vi "open.vi"(8 "error in (no error)":errorcluster, 11 "Scintilla window ref":refnum<k24>) -> (0 "error out":errorcluster, 3 "ScintillaNET out":refnum<class "ScintillaNET.lvclass">)   [LabVIEW 2018, in "ScintillaNET.lvclass"]
uses:
  ScintillaNET.lvclass
  D:/project/hobby/LF2R/LabVIEW/source/ScintillaNET/dll/ScintillaNET.dll
  dll/ScintillaNET.dll
  ScintillaNET.lvclass/ScintillaNET.ctl
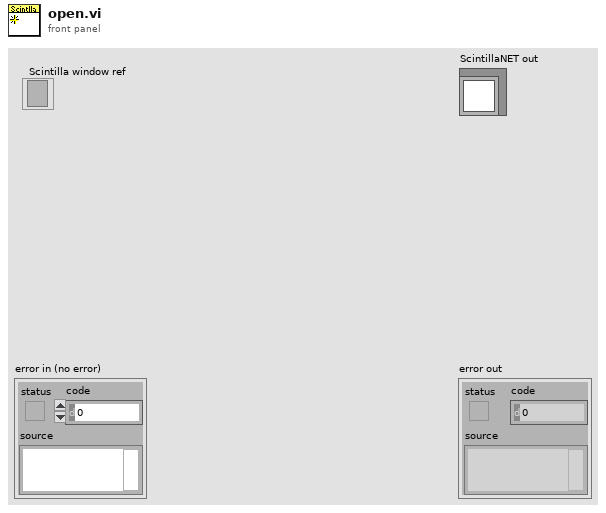
[diagram p1: front panel]
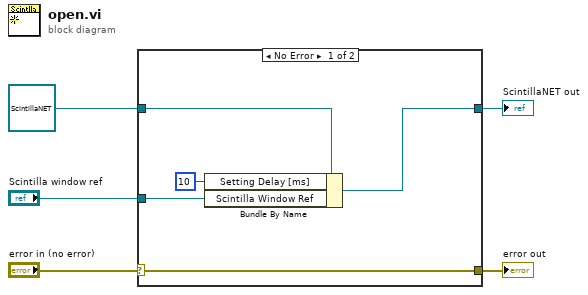
[diagram p0: block diagram]
diagram:
  n1 = case shown="No Error" "error in (no error)" {
    selector: "error in (no error)" -> [w9 w12]
    tunnel: [w9 w12] -> w4
    tunnel: [w8 w11] -> w2
    tunnel: refnum<class "ScintillaNET.lvclass"> refnum ("ScintillaNET in") -> [w10 w11]
    tunnel: "Scintilla window ref" -> [w7 _]
    frame No Error {
      n2 = Bundle By Name(cluster=w10, "Setting Delay [ms]"=u32 10, "Scintilla Window Ref"=w7) -> (w8:refnum<class "ScintillaNET.lvclass">)
    }
    frame Error {
    }
  }
  "error out" <- w4
  "ScintillaNET out" <- w2
